vi "Get Pot Zero.vi"() -> (2 "Left Pot 0":dbl, 3 "Right Pot 0":dbl)   [LabVIEW 2015]
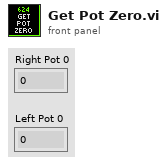
[diagram p1: front panel]
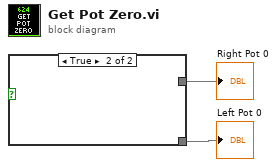
[diagram p0: block diagram]
diagram:
  n1 = case shown="True" {
    selector: _ -> [_ _]
    tunnel: [_ _] -> w2
    tunnel: [_ _] -> w1
    frame False {
    }
    frame True {
    }
  }
  "Right Pot 0" <- w2
  "Left Pot 0" <- w1
